vi "Error Handler.vi"(8 "error in (no error)":errorcluster) -> (0 "error out":errorcluster)   [LabVIEW 2020, in "Message Maker.lvlib"]
uses:
  Message Maker.lvlib
  <vilib>/Utility/error.llb/DialogType.ctl
panel:
  in  "Error Messages":string[](array[string])=["The message was created and added to your actor's library, but the changes to the library could not be saved because the actor contains an untitled VI.  Save or remove this VI, and then save the changes to your library.", "The message template library is locked, probably because it is in memory.  Remove the library from memory and try again.", "Selected parent class is not a Message.lvclass.  Select a different parent class.", "Target method name duplicates parent class name.", "A class or class folder with that name already exists.", "At least one of the selected VIs is not an actor public method.  No messages were created for these VIs.", "One or more attributes of the parent message class cannot be matched to an input of the target method.  You will need to complete the Do method manually.  Wire the output of Read Attributes.vi to the appropriate inputs of the actor's method.", "Message prototype has more than 6 controls.", "Rescripting failed. There are zero class constants on the block diagram of Do.vi. This makes it impossible to infer which class this message is intended for. You will need to edit this message class by hand.", "Target method not found.  Verify the message name matches a method of the target actor.", "At least one VI of the selected actor(s) is not a public method.  No messages were created for these VIs.", "This target depends on multiple Actor Framework libraries.  Only one library is allowed.  You must remove the extra dependencies before proceeding.", "Rescripting failed. There are multiple class constants on the block diagram of Do.vi. This makes it impossible to infer which class this message is intended for. You will need to edit this message class by hand."]
  in  "Error Codes":i32[](array[numeric])=[1019, 1562, 6001, 6002, 6003, 6004, 6005, 6006, 6007, 6008, 6009, 6010, 6011]
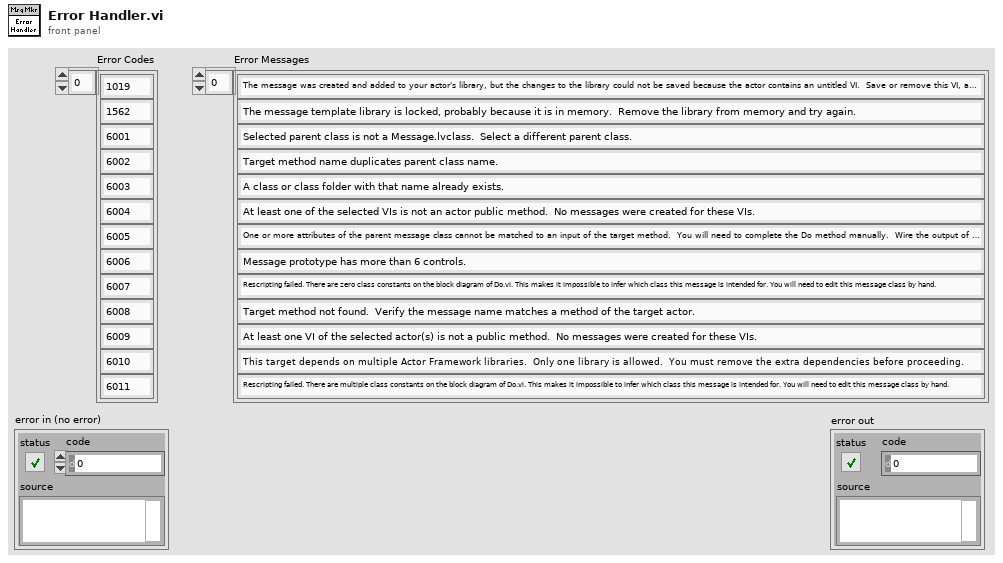
[diagram p1: front panel]
types:
  T1 = typedef "DialogType.ctl" = u16
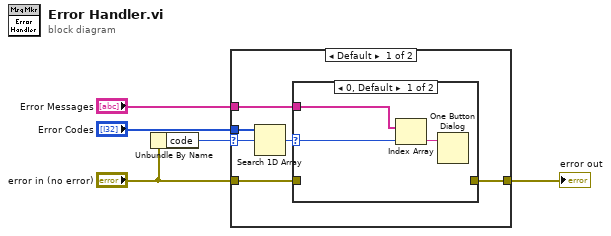
[diagram p0: block diagram]
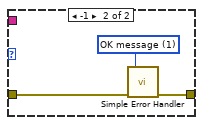
[diagram p2: hidden frame]
diagram:
  n1 = Unbundle By Name("error in (no error)") -> ("code"=w1:i32)
  n2 = case shown="Default" w1 {
    selector: w1 -> [w6 _]
    tunnel: "Error Codes" -> [w11 _]
    tunnel: "Error Messages" -> [w9 _]
    tunnel: "error in (no error)" -> [w8 w18]
    tunnel: [w7 w18] -> w2
    frame Default {
      n3 = Search 1D Array(1D array=w11, element=w6) -> (index of element=w10:i32)  [unwired: 1 in]
      n4 = case shown="0, Default" w10 {
        selector: w10 -> [w13 _]
        tunnel: w9 -> [w14 _]
        tunnel: w8 -> [_ w17]
        tunnel: [_ w16] -> w7
        frame 0, Default {
          n5 = Index Array(array=w14, index=w13) -> (element=w12:string)
          n6 = One Button Dialog(message=w12) -> ()  [unwired: 1 in, 1 out]
        }
        frame -1 {
          w15 = T1 1 items=["no dialog", "OK message", "continue or stop message", "OK message + warnings", "continue/stop + warnings"] ("type of dialog (OK msg:1)")
          n7 = call <vilib>:"Simple Error Handler.vi"("type of dialog (OK msg:1)"=w15, "error in (no error)"=w17) -> ("error out"=w16:errorcluster)  [unwired: 3 in, 4 out]
        }
      }
    }
    frame 43 {
      # "Ignore Operation Cancelled\nBy User"
    }
  }
  "error out" <- w2
